vi "Dequeue Cmds From Nodes.vi"(6 "Ready For Output?":bool, 7 "NumNodes":u8=1, 8 "error in":errorcluster, 11 "Communication FIFOs":T2={"FIFOs.Node 0"={"SendCmdFIFO"="", "ReceiveDataFIFO"=""}, "FIFOs.Node 1"={"SendCmdFIFO"="Bus0_Dev0_Ch0_TxFIFO", "ReceiveDataFIFO"=""}, "FIFOs.Node 2"={"SendCmdFIFO"="Bus0_Dev0_Ch0_TxFIFO", "ReceiveDataFIFO"=""}, "FIFOs.Node 3"={"SendCmdFIFO"="Bus0_Dev0_Ch0_TxFIFO", "ReceiveDataFIFO"=""}, "FIFOs.Node 4"={"SendCmdFIFO"="Bus0_Dev0_Ch0_TxFIFO", "ReceiveDataFIFO"=""}}) -> (0 "error out":errorcluster, 1 "Cmd Received Valid":bool, 2 "Cmd Received":T1, 5 "Current Node":u8)   [LabVIEW 2014, in "IO Node Logic Template_SPIBus0.lvlib"]
uses:
  IO Node Logic Template_SPIBus0.lvlib
  Controls/All Nodes Resources.ctl
  Node/Controls/NodeResources FIFOs.ctl
  Node/Controls/Node_Command_Sent.ctl
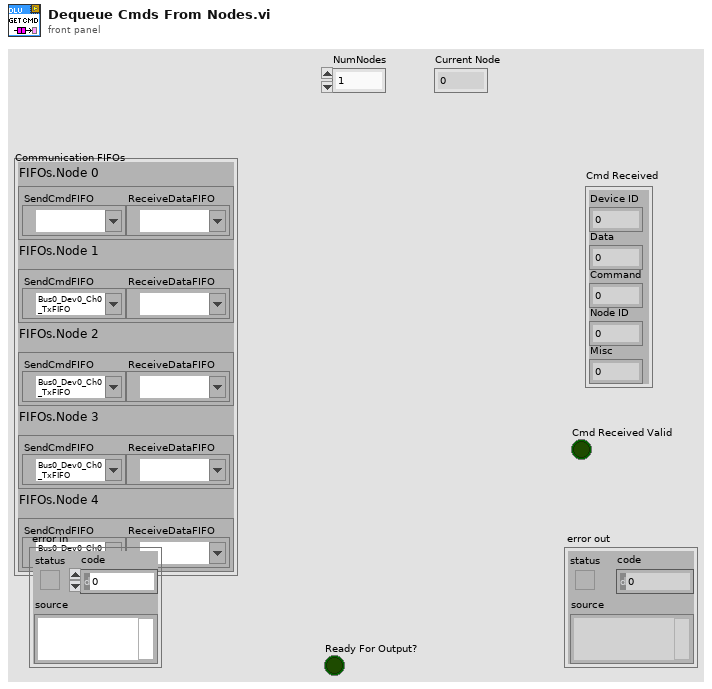
[diagram p1: front panel]
types:
  T1 = typedef "IO Node Logic Template_SPIBus0.lvlib/Node_Command_Sent.ctl" = cluster{"Device ID":u8, "Data":u64, "Command":u8, "Node ID":u8, "Misc":u8}
  T2 = typedef "IO Node Logic Template_SPIBus0.lvlib/All Nodes Resources.ctl" = cluster{"FIFOs.Node 0":T3, "FIFOs.Node 1":T3, "FIFOs.Node 2":T3, "FIFOs.Node 3":T3, "FIFOs.Node 4":T3}
  T3 = typedef "IO Node Logic Template_SPIBus0.lvlib/NodeResources FIFOs.ctl" = cluster{"SendCmdFIFO":refnum<k21>, "ReceiveDataFIFO":refnum<k21>}
  T4 = cluster{"Channel ID":u8, "Data":u64, "Command":u8, "Sender Address":u8, "Misc":u8}
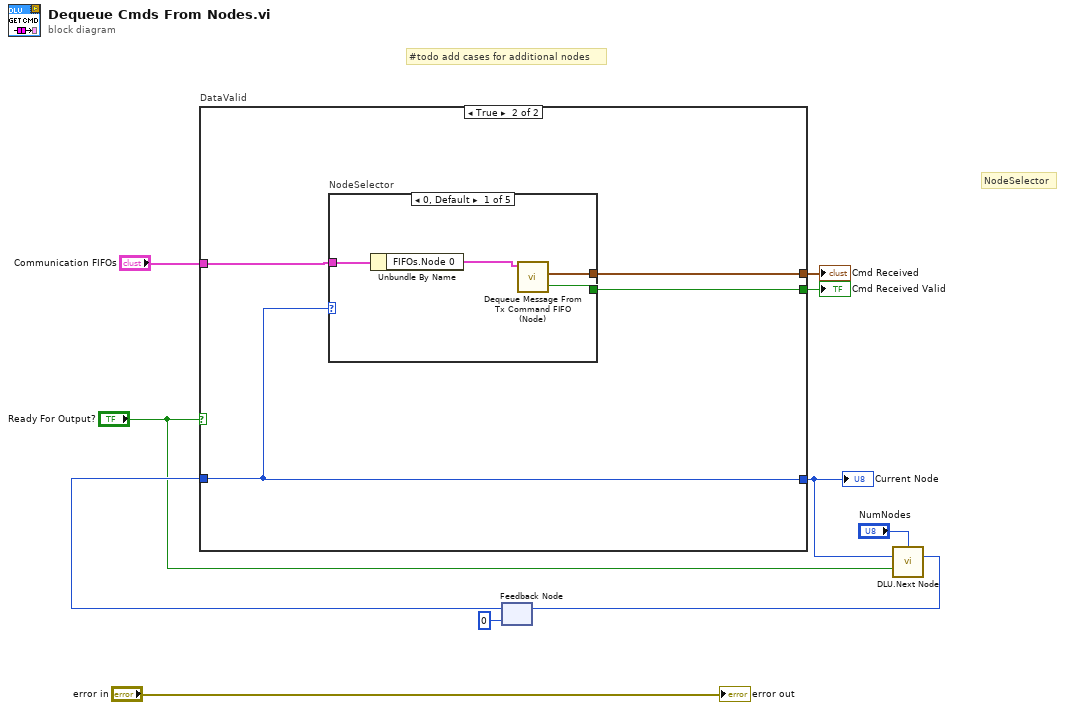
[diagram p0: block diagram]
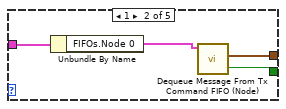
[diagram p3: hidden frame]
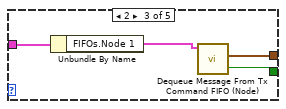
[diagram p4: hidden frame]
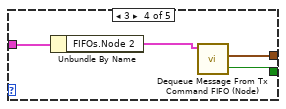
[diagram p5: hidden frame]
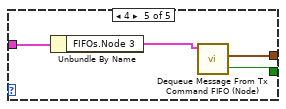
[diagram p6: hidden frame]
diagram:
  # "#todo add cases for additional nodes"
  # "NodeSelector"
  n1 = feedback #1(u8 0 ("Next Node")) -> (w7:u8)
  n2 = case "DataValid" shown="True" "Ready For Output?" {
    tunnel: w7 -> [w11 w12]
    tunnel: "Communication FIFOs" -> [_ w15]
    tunnel: [_ w14] -> w3
    tunnel: [_ w13] -> w2
    tunnel: [w11 w12] -> w6
    frame False {
    }
    frame True {
      n3 = case "NodeSelector" shown="0, Default" w12 {
        tunnel: w15 -> [w19 w23 w27 w31 w35]
        tunnel: [w18 w22 w26 w30 w34] -> w14
        tunnel: [w17 w21 w25 w29 w33] -> w13
        frame 0, Default {
          n4 = Unbundle By Name(w19) -> ("FIFOs.Node 0"=w16:T3)
          n5 = call "Dequeue Message From Tx Command FIFO (Node).vi"("FIFOs: I/O Node"=w16) -> ("Cmd Received Valid"=w17:bool, "Cmd Received"=w18:T4)  [unwired: 7 in, 2 out]
        }
        frame 1 {
          n6 = Unbundle By Name(w23) -> ("FIFOs.Node 0"=w20:T3)
          n7 = call "Dequeue Message From Tx Command FIFO (Node).vi"("FIFOs: I/O Node"=w20) -> ("Cmd Received Valid"=w21:bool, "Cmd Received"=w22:T4)  [unwired: 7 in, 2 out]
        }
        frame 2 {
          n8 = Unbundle By Name(w27) -> ("FIFOs.Node 1"=w24:T3)
          n9 = call "Dequeue Message From Tx Command FIFO (Node).vi"("FIFOs: I/O Node"=w24) -> ("Cmd Received Valid"=w25:bool, "Cmd Received"=w26:T4)  [unwired: 7 in, 2 out]
        }
        frame 3 {
          n10 = Unbundle By Name(w31) -> ("FIFOs.Node 2"=w28:T3)
          n11 = call "Dequeue Message From Tx Command FIFO (Node).vi"("FIFOs: I/O Node"=w28) -> ("Cmd Received Valid"=w29:bool, "Cmd Received"=w30:T4)  [unwired: 7 in, 2 out]
        }
        frame 4 {
          n12 = Unbundle By Name(w35) -> ("FIFOs.Node 3"=w32:T3)
          n13 = call "Dequeue Message From Tx Command FIFO (Node).vi"("FIFOs: I/O Node"=w32) -> ("Cmd Received Valid"=w33:bool, "Cmd Received"=w34:T4)  [unwired: 7 in, 2 out]
        }
      }
    }
  }
  "Cmd Received" <- w3
  "Cmd Received Valid" <- w2
  "Current Node" <- w6
  n14 = call "DLU.Next Node.vi"("NumNodes"="NumNodes", "Current Node"=w6, "Move to Next Node"="Ready For Output?") -> ("Next Node"=w9:u8)  [unwired: 12 in]
  n15 = feedback-in #1(w9) -> ()
  "error out" <- "error in"
